vi "TempMeasOneSetZ.vi"(0 "meas_setting":T1 {"zStartDistCm" format="%.2f"; "numTxCycles" format="%.1f"; "profTxVoltageVolt" format="%#_1g"; "ceilTxVoltageVolt" format="%.2f"; "maxTxVoltageVolt" format="%.2f"; "focusRangeCm" format="%.1f"; "txFrequencyHz" format="%.2f"}, 1 "Comment(SN)":string, 2 "CW":bool, 5 "initial \ncommand":bool=TRUE, 7 "Database":T2, 9 "Z Address":T3, 11 "error in (no error)":errorcluster, 12 "Log file":path=path "nologfile") -> (15 "error out":errorcluster)   [LabVIEW 2016]
doc: "This program sets up runs one complete intensity measurement and voltage-dependent measurements. It calls subroutines to get hydrophone sensitivity, set Z system transmit parameters via Telnet, run the intensity measurement, and check the data. Next, the voltage-dependent measurement is made and checked. The data is saved to the database (or to a local file if errors have been found) and the results are printed. The program returns the result ID from the database, and any warnings or errors found."
uses:
  type def/ZAddress.ctl
  type def/Database.ctl
  type def/measSetting.ctl
  user/GrobaLimitVoltage.vi
  TemperatureMeasure/Thermal_type.vi
panel:
  in  "ScanRange coeff for PRF":dbl[][](array[numeric])=[[2.5, 1.6, 1.2, 1.0, 0.8], [2.3, 1.6, 1.2, 1.0, 0.8], [1.9, 1.6, 1.2, 1.0, 0.8], [1.7, 1.5, 1.2, 1.0, 0.8], [1.6, 1.4, 1.2, 1.0, 0.8]]
  out "Receive array":string[](array[string])=["\r\n220 OK\r\nContainers within Hardware Control Layer\r\n\tHardwareModel\r\n\tHardwareControl\r\n\tHardwareAlgorithm\r\n\tSeq\r\n\tBeamforming\r\n\tDigitalReceiver\r\n\tEchoProcessor\r\n\tFlowProcessor\r\n\tHardwareScanConverter\r\n\tSip\r\n\tVideoInterface\r\n\tRtc\r\n\tCine\r\nScalar Parameters of Hardware Control Layer\r\nArray Parameters of Hardware Control Layer\r\ndebug\tDebug Functions\r\nquit\tExit DIOS\r\nback\tPrevious menu\r\nmain\tTop menu\r\nhelp\tAvailable commands\r\n\r\n", "\r\n220 OK\r\nContainers within Beamforming\r\n\tCommon\r\n\tBImage\r\n\tCbImage\r\n\tDImage\r\nScalar Parameters of Beamforming\r\nArray Parameters of Beamforming\r\ndebug\tDebug Functions\r\nquit\tExit DIOS\r\nback\tPrevious menu\r\nmain\tTop menu\r\nhelp\tAvailable commands\r\n\r\n", "\r\n220 OK\r\nContainers within Common\r\nScalar Parameters of Common\r\n\tBfPropagationVelCmPerSec\t154000\r\n\tDisUnit\t0.00385\r\n\tHwRcInterruptMask\t63\r\n\tHwRcTVP\t3\r\n\tHwRxAac0\t175\r\n\tHwRxAac1\t0\r\n\tHwRxbfBlankingWord\t0\r\n\tHwRxbfCmd1Word\t4232\r\n\tHwRxbfCmd2Word\t2\r\n\tHwRxbf0Cmd2Word\t3\r\n\tHwRxbfStartDelayWord\t10\r\n\tHwTiAttenuatorSelect\t0\r\n\tHwTiBitEn\t25088\r\n\tHwTiDacCtrl0\t255\r\n\tHwTiDacCtrl1\t2303\r\n\tHwTiDacCtrl2\t3327\r\n\tHwTiDacCtrl3\t511\r\n\tHwTiDacCtrl4\t2559\r\n\tHwTiDacCtrl5\t3583\r\n\tHwTiDacCtrl6\t767\r\n\tHwTiDacCtrl7\t2815\r\n\tHwTiDacCtrl8\t3839\r\n\tHwTiDacCtrl9\t2047\r\n\tHwTiDacCtrl10\t4095\r\n\tHwTiDigitalDriveCtrl\t0\r\n\tHwTiDigitalInterruptPolarity\t0\r\n\tHwTiDigitalReadCtrl\t0\r\n\tHwTiEchoBoosterCtrl\t0\r\n\tHwTiGlobalCtrl\t1\r\n\tHwTiHighVoltEn\t0\r\n\tHwTiInterruptClear\t65535\r\n\tHwTiInterruptMask\t32767\r\n\tHwTiMiscBitCtrl\t12\r\n\tHwTiProbeSelect\t2\r\n\tHwTiTXCLTransfer\t0\r\n\tHwTiVoltMultiplexer\t0\r\n\tHwTrGlobalCtrlAll\t1\r\n\tHwTrGlobalCtrl0All\t0\r\n\tHwTrDiagnosticCtrlAll\t0\r\n\tHwTrInterruptMaskAll\t1\r\n\tHwTrInterruptClearAll\t1\r\n\tHwTrRealTimeCtrlAll\t40\r\n\tHwTrTgcAacSignalCtrlAll\t0\r\n\tRxDelayRefx\t1\r\n\tRxDelayRefy\t-1\r\n\tTrPartNumber\t5928150\r\n\tBfPropagationVelFactor\t1\r\n\tDigitizingRateHz\t4e+007\r\n\tHwRxBfVectorLengthWord\t0\r\n\tIsRxVectorLengthEn\t1\r\n\tNumChannels\t192\r\n\tProbeBandwidthHz\t3.6e+006\r\n\tProbeId\t171\r\n\tProbeNumElem\t192\r\n\tProbeNumRows\t1\r\n\tProbePitchCm\t0.02\r\n\tProbeRadiusElectricalCm\t0\r\n\tProbeType\t0\r\n\tPropagationVelCmPerSec\t154000\r\n\tRxApod2dEn\t0\r\n\tRxbfAdcDelayClocks\t10\r\n\tRxbfGainShift\t0\r\n\tRxDelayYOffsetSysClk4\t0\r\n\tTxPulserMaxVolt\t50\r\nArray Parameters of Common\r\n\tHwRxbf0AdGainA\tsize=64\r\n\tHwRxbf1AdGainA\tsize=64\r\n\tHwRxbf2AdGainA\tsize=64\r\n\tHwRxbf3AdGainA\tsize=64\r\n\tHwRxbf4AdGainA\tsize=64\r\n\tHwRxbf5AdGainA\tsize=64\r\n\tHwRxbf6AdGainA\tsize=64\r\n\tHwRxbf7AdGainA\tsize=64\r\n\tHwRxbf8AdGainA\tsize=64\r\n\tHwRxbf9AdGainA\tsize=64\r\n\tHwRxbf10AdGainA\tsize=64\r\n\tHwRxbf11AdGainA\tsize=64\r\n\tHwRxAdOffsetCalA\tsize=192\r\n\tHwRxApodFilterRamA\tsize=512\r\n\tHwRxbf0DelayCalA\tsize=64\r\n\tHwRxbf1DelayCalA\tsize=64\r\n\tHwRxbf2DelayCalA\tsize=64\r\n\tHwRxbf3DelayCalA\tsize=64\r\n\tHwRxbf4DelayCalA\tsize=64\r\n\tHwRxbf5DelayCalA\tsize=64\r\n\tHwRxbf6DelayCalA\tsize=64\r\n\tHwRxbf7DelayCalA\tsize=64\r\n\tHwRxbf8DelayCalA\tsize=64\r\n\tHwRxbf9DelayCalA\tsize=64\r\n\tHwRxbf10DelayCalA\tsize=64\r\n\tHwRxbf11DelayCalA\tsize=64\r\n\tHwRxbf0DxA\tsize=64\r\n\tHwRxbf1DxA\tsize=64\r\n\tHwRxbf2DxA\tsize=64\r\n\tHwRxbf3DxA\tsize=64\r\n\tHwRxbf4DxA\tsize=64\r\n\tHwRxbf5DxA\tsize=64\r\n\tHwRxbf6DxA\tsize=64\r\n\tHwRxbf7DxA\tsize=64\r\n\tHwRxbf8DxA\tsize=64\r\n\tHwRxbf9DxA\tsize=64\r\n\tHwRxbf10DxA\tsize=64\r\n\tHwRxbf11DxA\tsize=64\r\n\tHwRxbf0DyA\tsize=64\r\n\tHwRxbf1DyA\tsize=64\r\n\tHwRxbf2DyA\tsize=64\r\n\tHwRxbf3DyA\tsize=64\r\n\tHwRxbf4DyA\tsize=64\r\n\tHwRxbf5DyA\tsize=64\r\n\tHwRxbf6DyA\tsize=64\r\n\tHwRxbf7DyA\tsize=64\r\n\tHwRxbf8DyA\tsize=64\r\n\tHwRxbf9DyA\tsize=64\r\n\tHwRxbf10DyA\tsize=64\r\n\tHwRxbf11DyA\tsize=64\r\n\tHwRxbf0DzA\tsize=128\r\n\tHwRxbf1DzA\tsize=128\r\n\tHwRxbf2DzA\tsize=128\r\n\tHwRxbf3DzA\tsize=128\r\n\tHwRxbf4DzA\tsize=128\r\n\tHwRxbf5DzA\tsize=128\r\n\tHwRxbf6DzA\tsize=128\r\n\tHwRxbf7DzA\tsize=128\r\n\tHwRxbf8DzA\tsize=128\r\n\tHwRxbf9DzA\tsize=128\r\n\tHwRxbf10DzA\tsize=128\r\n\tHwRxbf11DzA\tsize=128\r\n\tHwRxbf0PosInApodWinA\tsize=64\r\n\tHwRxbf1PosInApodWinA\tsize=64\r\n\tHwRxbf2PosInApodWinA\tsize=64\r\n\tHwRxbf3PosInApodWinA\tsize=64\r\n\tHwRxbf4PosInApodWinA\tsize=64\r\n\tHwRxbf5PosInApodWinA\tsize=64\r\n\tHwRxbf6PosInApodWinA\tsize=64\r\n\tHwRxbf7PosInApodWinA\tsize=64\r\n\tHwRxbf8PosInApodWinA\tsize=64\r\n\tHwRxbf9PosInApodWinA\tsize=64\r\n\tHwRxbf10PosInApodWinA\tsize=64\r\n\tHwRxbf11PosInApodWinA\tsize=64\r\n\tHwRxMuxSelectLutA\tsize=512\r\n\tHwRxRamOffsetA\tsize=12\r\n\tHwTxDacA\tsize=2\r\n\tHwTxpgDelayAperA\tsize=393216\r\n\tNumBitsPerCycleA\tsize=49\r\n\tNumCyclesPerPassA\tsize=49\r\n\tNumWordsPerPassA\tsize=49\r\n\tRxAdGainA\tsize=256\r\n\tRxDelayCalA\tsize=768\r\n\tRxDxA\tsize=256\r\n\tRxDyA\tsize=256\r\n\tRxDzA\tsize=256\r\n\tRxMuxSelectLutPtrA\tsize=512\r\n\tRxPosInApodWinA\tsize=768\r\n\tTxDelayCalA\tsize=192\r\n\tTxpgWaveformHoutA\tsize=15680\r\n\tTxpgWaveformLoutA\tsize=15680\r\n\tYIndexTableA\tsize=256\r\n\tZIndexTableA\tsize=256\r\n\tInsertedProbeIdA\tsize=6\r\n\tPulseVoltageA\tsize=2\r\n\tRxApodFactorA\tsize=4\r\n\tRxApodSelA\tsize=4\r\n\tSysTxFreqHzA\tsize=49\r\ndebug\tDebug Functions\r\nquit\tExit DIOS\r\nback\tPrevious menu\r\nmain\tTop menu\r\nhelp\tAvailable commands\r\n\r\n", "220 OK\r\n", "250 20\r\n"]
  out "ProbeType":i8
  out "PID PRF":dbl format="%#.2f"
  out "error out 2":errorcluster caption="error out"
  out "size(s)":i32
  out "min Array":dbl[](array[numeric]) format="%.2f"
  out "Span Array":dbl[](array[numeric]) format="%.2f"
  out "TxElement array":i32[](array[numeric])
  out "Large RoiMin":dbl
  out "Large RoiSpan":dbl
  out "Small TxElement":i32
  in  "connection ID":refnum<k5>
  in  "tcp timeout (sec)":sgl=40.0 format="%.2f"
  in  "z tolCm":sgl=0.005 format="%.3f"
  # "Program constants"
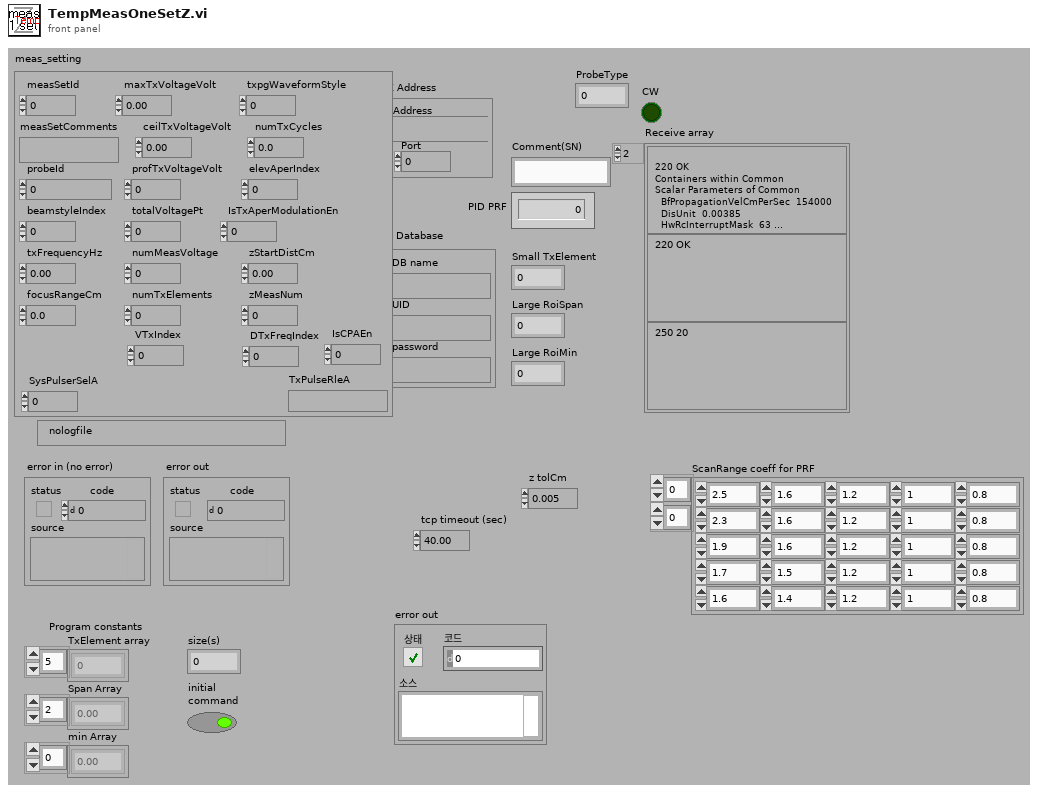
[diagram p1: front panel]
types:
  T1 = typedef "measSetting.ctl" = cluster{"measSetId":i32, "measSetComments":string, "probeId":sgl, "beamstyleIndex":i16, "txFrequencyHz":sgl, "focusRangeCm":sgl, "maxTxVoltageVolt":sgl, "ceilTxVoltageVolt":sgl, "profTxVoltageVolt":dbl, "totalVoltagePt":i8, "numMeasVoltage":i8, "numTxElements":i16, "txpgWaveformStyle":i8, "numTxCycles":sgl, "elevAperIndex":i8, "zStartDistCm":sgl, "zMeasNum":i8, "IsTxAperModulationEn":i8, "DTxFreqIndex":i16, "VTxIndex":i8, "IsCPAEn":i16, "SysPulserSelA":i16, "TxPulseRleA":string}
  T2 = typedef "Database.ctl" = cluster{"DB name":string, "UID":string, "password":string}
  T3 = typedef "ZAddress.ctl" = cluster{"Address":string, "Port":u16}
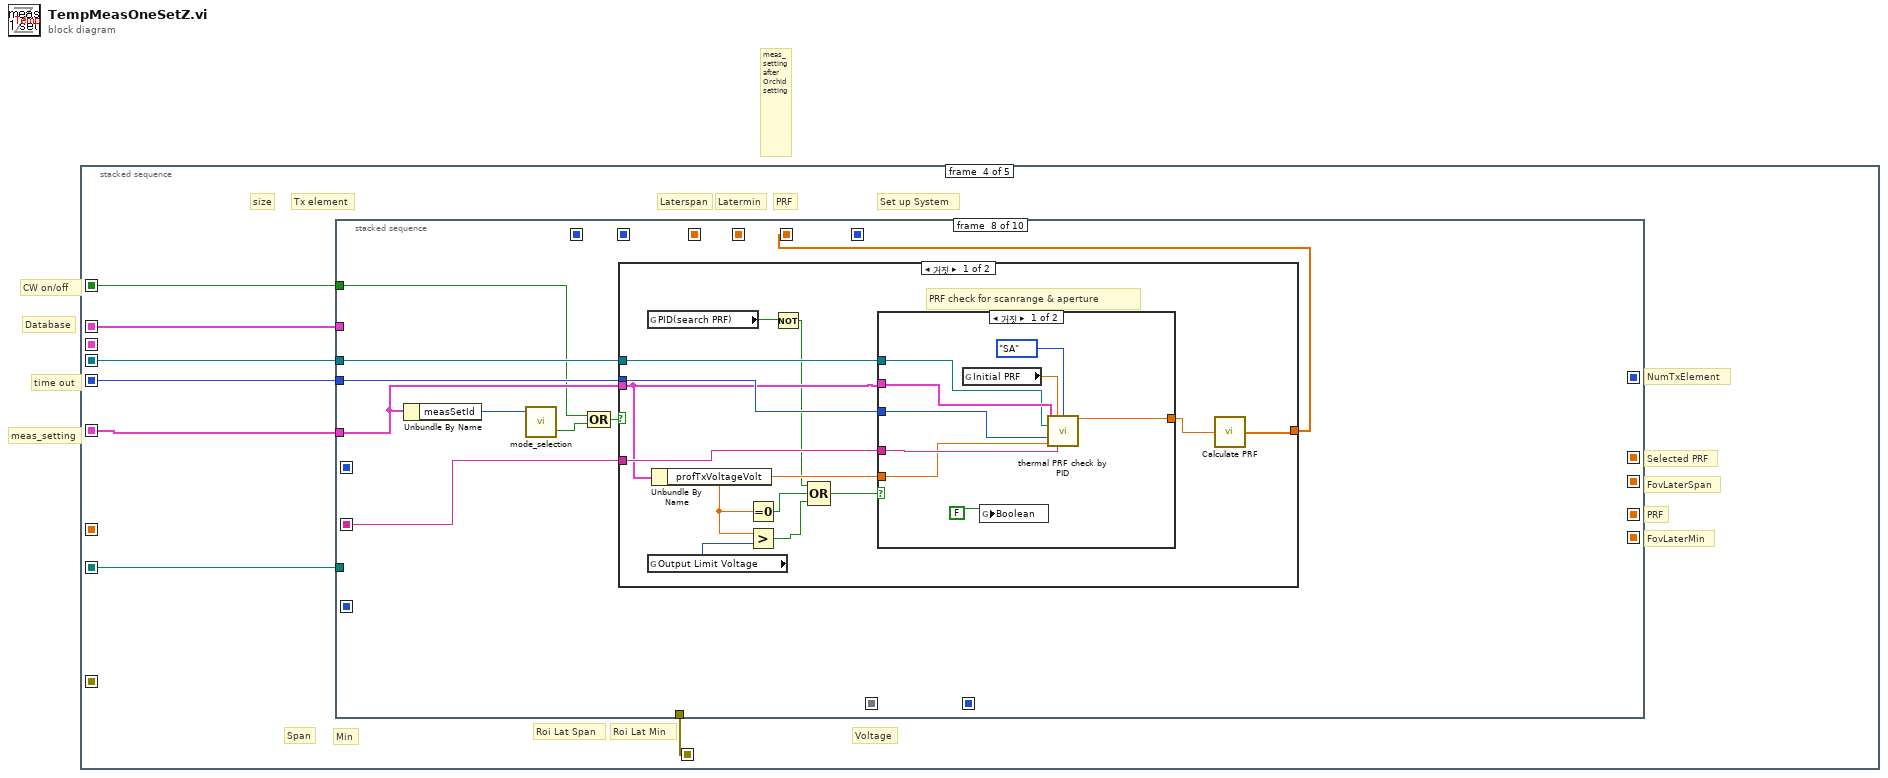
[diagram p0: block diagram]
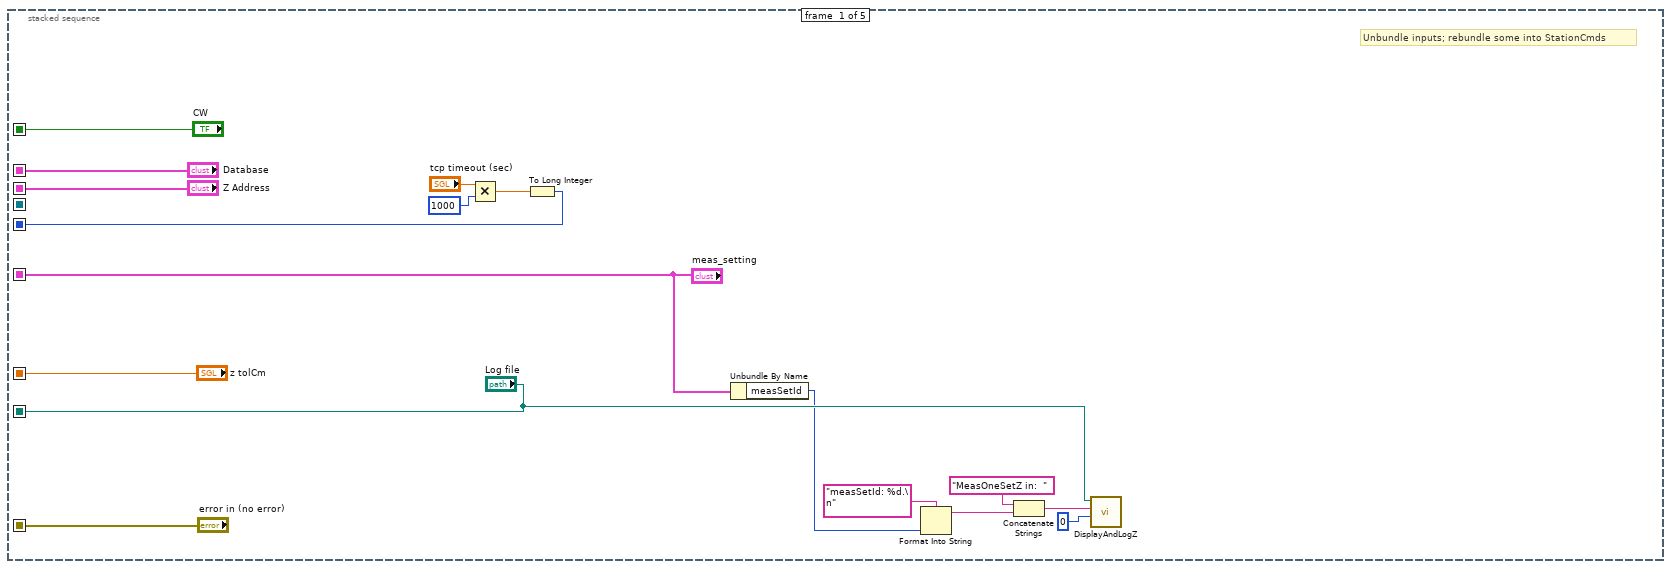
[diagram p2: hidden frame]
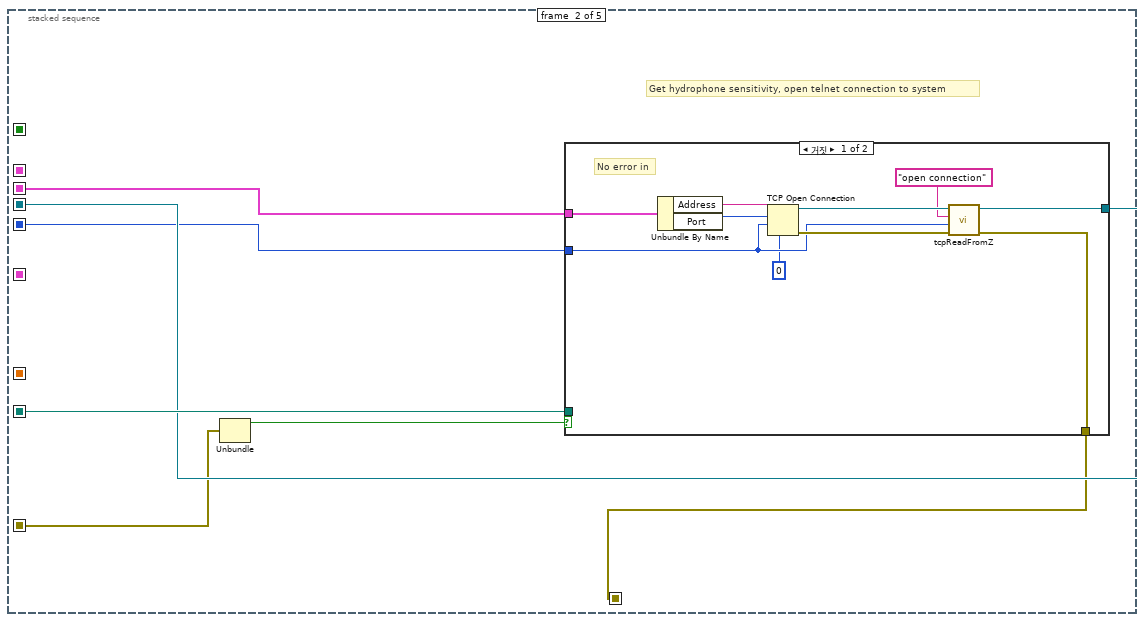
[diagram p3: hidden frame]
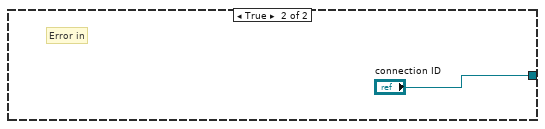
[diagram p4: hidden frame]
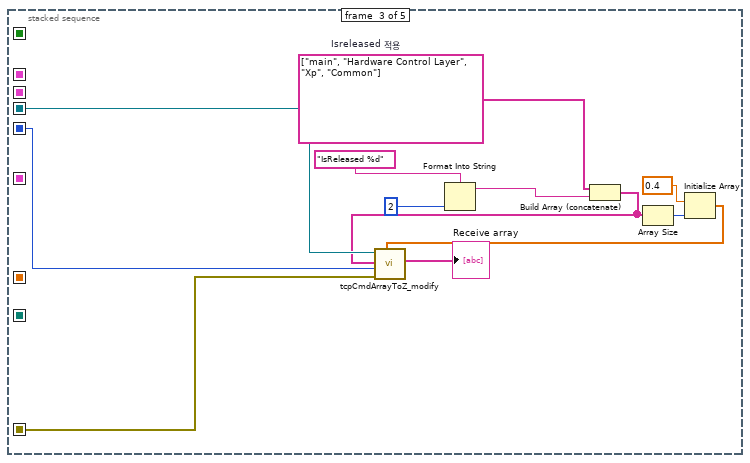
[diagram p5: hidden frame]
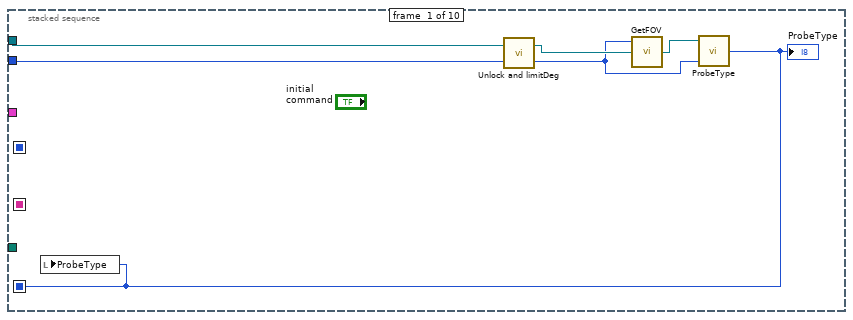
[diagram p6: hidden frame]
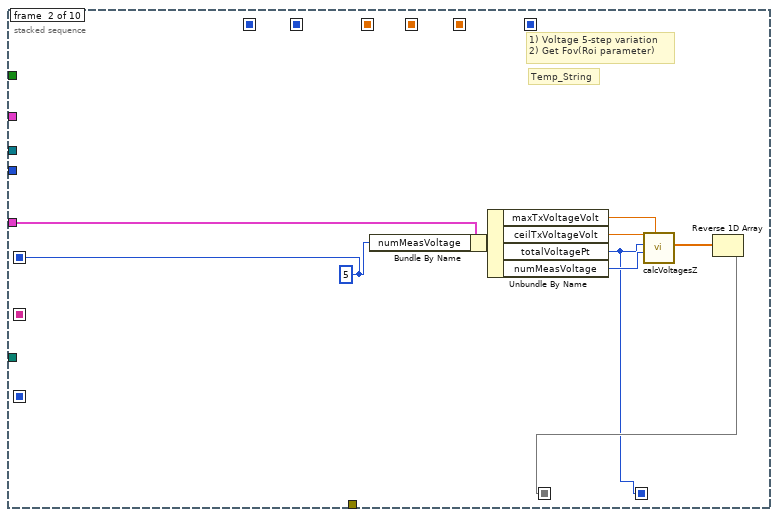
[diagram p7: hidden frame]
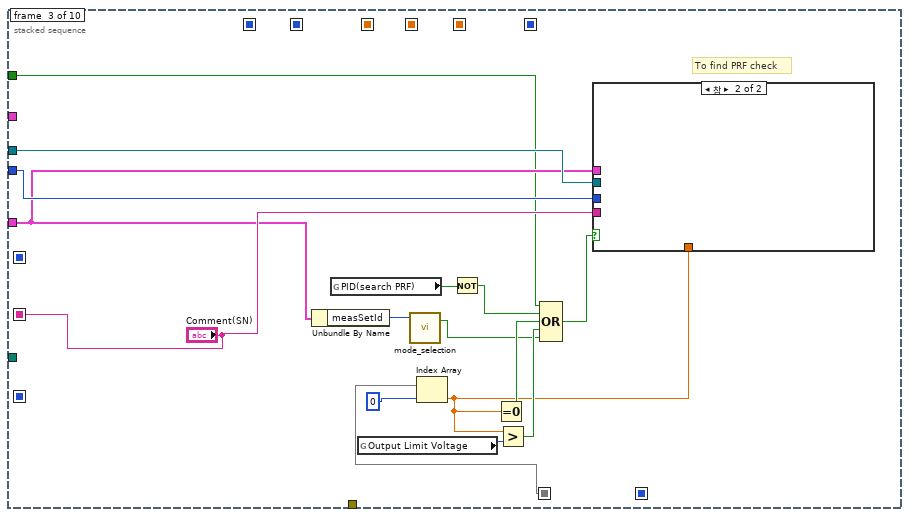
[diagram p8: hidden frame]
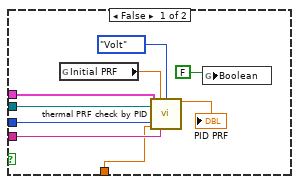
[diagram p9: hidden frame]
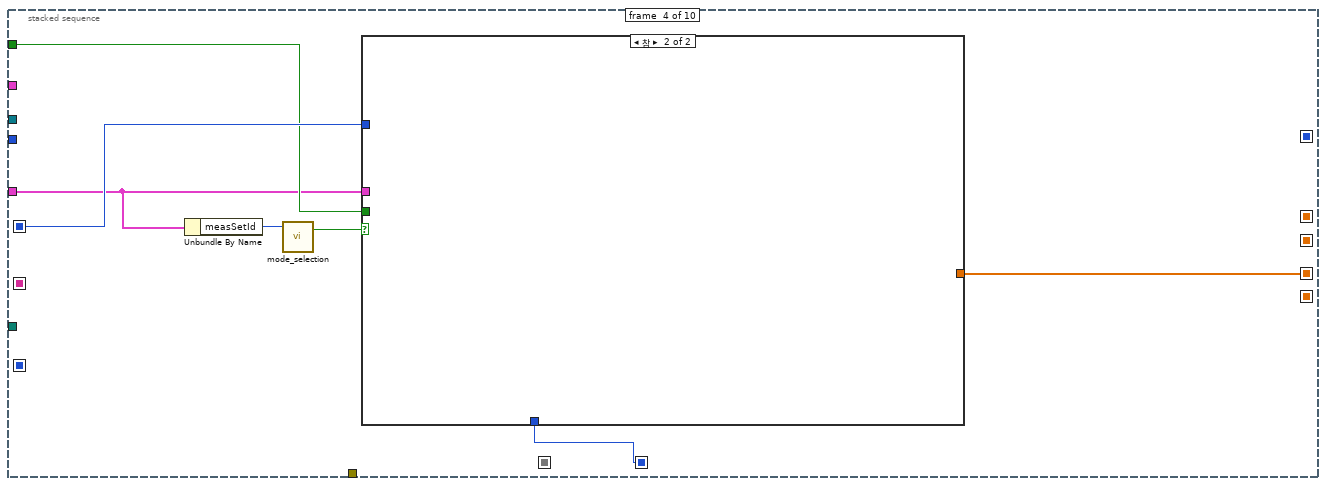
[diagram p10: hidden frame]
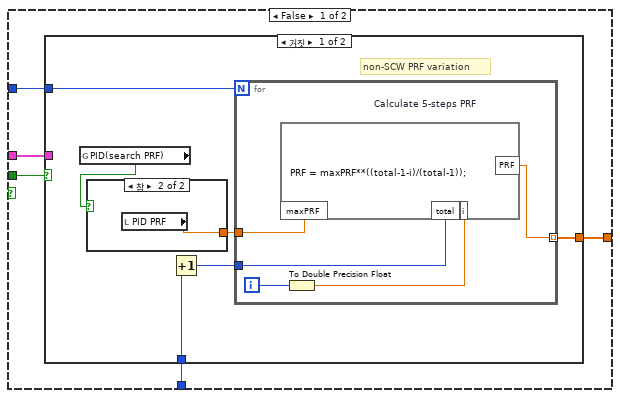
[diagram p11: hidden frame]
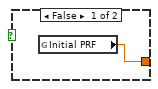
[diagram p12: hidden frame]
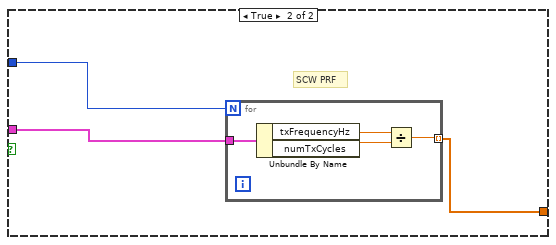
[diagram p13: hidden frame]
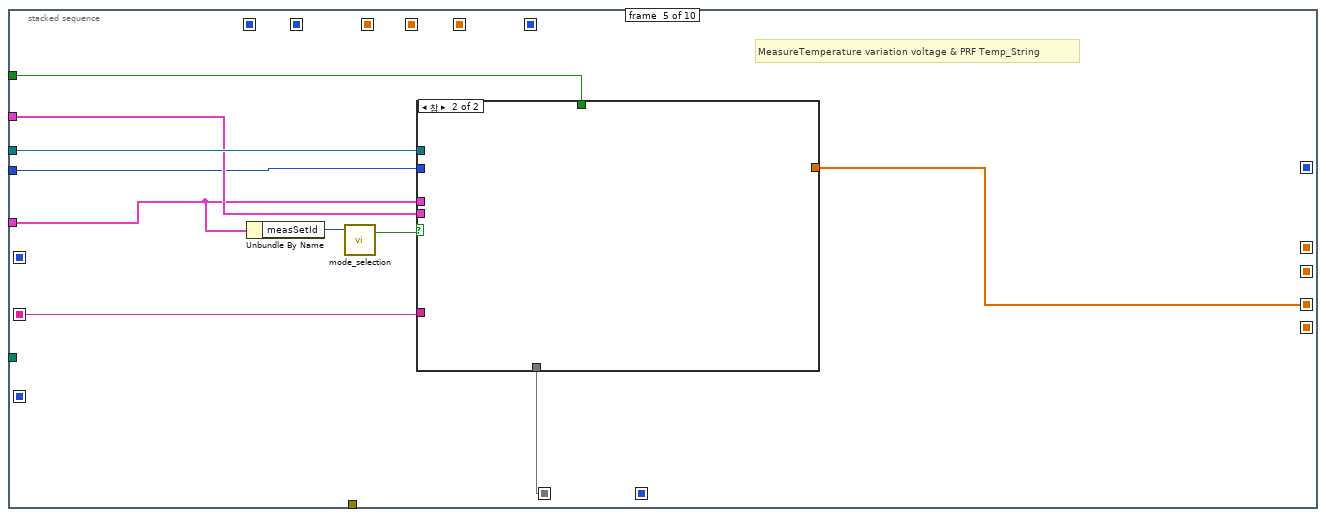
[diagram p14: hidden frame]
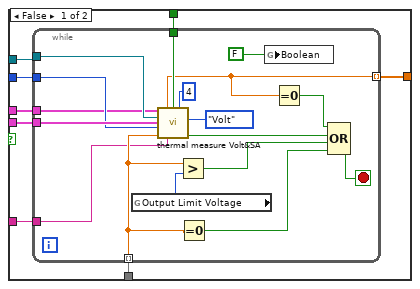
[diagram p15: hidden frame]
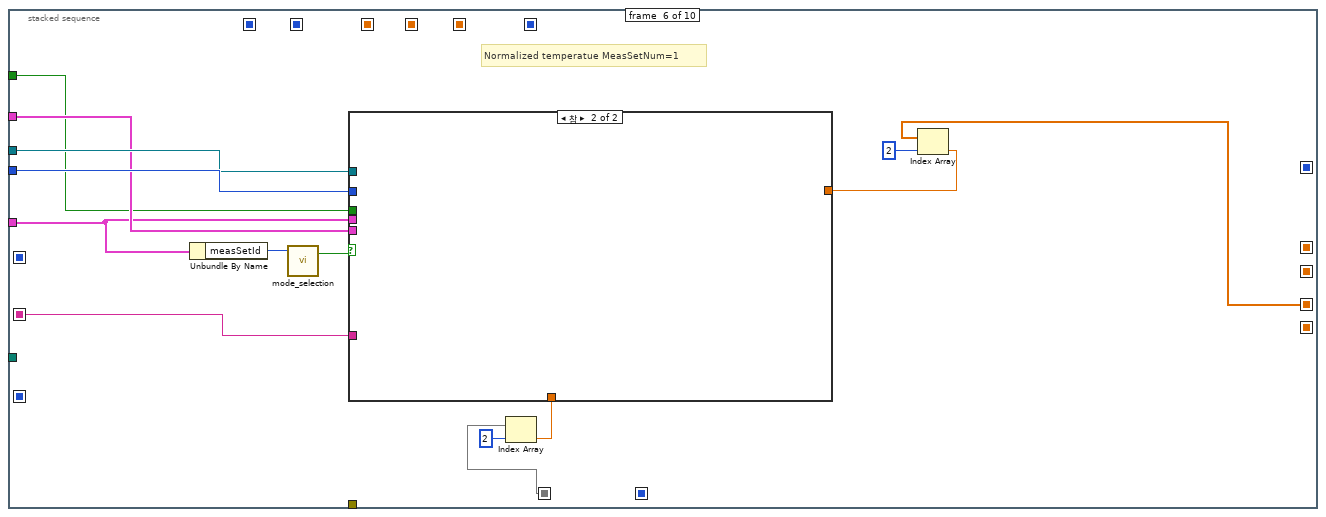
[diagram p16: hidden frame]
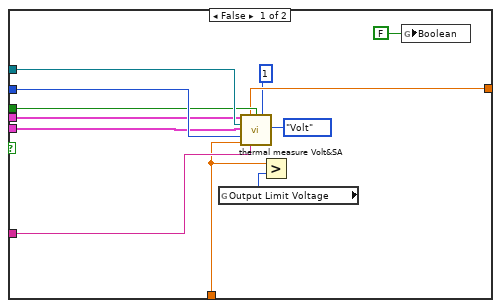
[diagram p17: hidden frame]
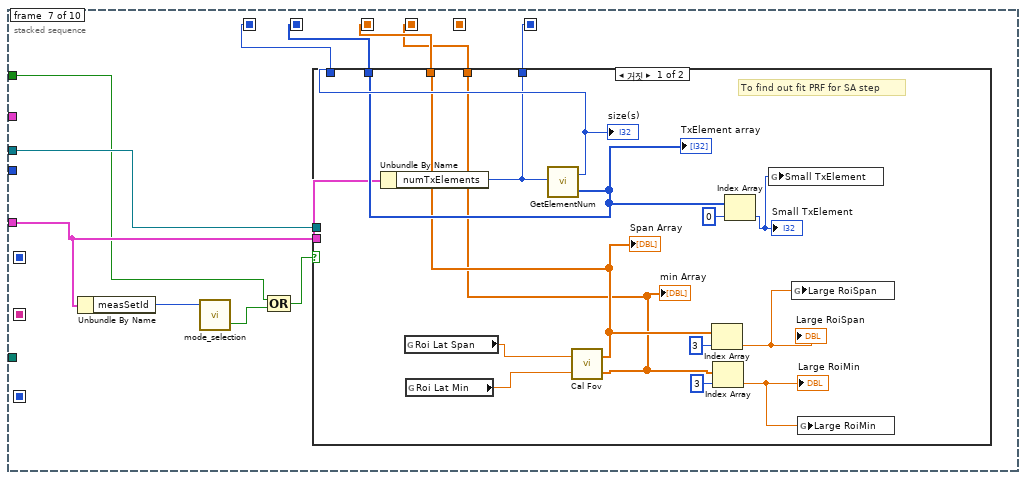
[diagram p18: hidden frame]
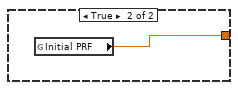
[diagram p20: hidden frame]
diagram:
  # "CW on/off"
  # "time out"
  # "Database"
  # "meas_setting"
  # "meas_setting\nafter Orchid setting"
  n1 = stacked-sequence {
    seq-local: ["Database" _ _ _ _] -> [_ _ _ w53 _]
    seq-local: ["Z Address" _ _ _ _] -> [_ w23 _ _ _]
    seq-local: ["Log file" _ _ _ _] -> [_ w24 _ w54 w372]
    seq-local: ["meas_setting" _ _ _ _] -> [_ _ _ w52 _]
    seq-local: ["z tolCm" _ _ _ _] -> [_ _ _ _ _]
    seq-local: [_ w21 _ _ _] -> [_ _ _ w48 w362]
    seq-local: [w5 _ _ _ _] -> [_ w20 w45 w50 w363]
    seq-local: [_ w22 _ _ _] -> [_ _ w47 w51 w364]
    seq-local: ["error in (no error)" _ _ _ _] -> [_ w19 w46 _ _]
    seq-local: ["CW" _ _ _ _] -> [_ _ _ w49 _]
    frame #0 {
      # "Unbundle inputs; rebundle some into StationCmds"
      n2 = Multiply(x="tcp timeout (sec)", y=i16 1000) -> (x*y=w6:sgl)
      n3 = To Long Integer(number=w6) -> (32bit integer=w5:i32)
      n4 = Unbundle By Name("meas_setting") -> ("measSetId"=w3:i32)
      n5 = Format Into String(format string="measSetId: %d.\n" ("Substring"), w3) -> (resulting string=w12:string)  [unwired: 2 in, 1 out]
      n6 = Concatenate Strings("MeasOneSetZ in:  " ("Substring"), w12) -> (w13:string)
      n7 = call "DisplayAndLogZ.vi"("Log file"="Log file", "message"=w13, "action (0: log+display)"=u16 0) -> ()  [unwired: 5 in, 1 out]
    }
    frame #1 {
      # "Get hydrophone sensitivity, open telnet connection to system"
      n8 = Unbundle(w19) -> ("status"=w18:bool)  [unwired: 2 out]
      n9 = case shown="거짓" w18 {
        tunnel: w24 -> [_ _]
        tunnel: w23 -> [w29 _]
        tunnel: [w28 "connection ID"] -> w22
        tunnel: [w26 _] -> w21
        tunnel: w20 -> [w27 _]
        frame False {
          # "No error in"
          n10 = Unbundle By Name(w29) -> ("Address"=w33:string, "Port"=w32:u16)
          n11 = TCP Open Connection(address=w33, remote port or service name=w32, timeout ms (60000)=w27, local port=u16 0) -> (connection ID=w31:refnum<k5>, error out=w34:errorcluster)  [unwired: 1 in]
          n12 = call "tcpReadFromZ.vi"("error in (no error)"=w34, "Timeout (40000 ms)"=w27, "Command sent"="open connection", "connection ID in"=w31) -> ("error out"=w26:errorcluster, "connection ID out"=w28:refnum<k5>)  [unwired: 3 in, 3 out]
        }
        frame True {
          # "Error in"
        }
      }
    }
    frame #2 {
      w38 = string[] ["main", "Hardware Control Layer", "Xp", "Common"]  # Isreleased 적용
      n13 = Format Into String(format string="IsReleased %d" ("Format String"), i16 2 ("입력 1")) -> (resulting string=w43:string)  [unwired: 2 in, 1 out]
      n14 = Build Array (concatenate)(w38, w43) -> (w40:string[])
      n15 = Array Size(array=w40) -> (size(s)=w42:i32)
      n16 = Initialize Array(0.4 ("element"), w42) -> (w39:dbl[])
      n17 = call "tcpCmdArrayToZ_modify.vi"("Delay (sec)"=w39, "error in (no error)"=w46, "Timeout (ms)"=w45, "Command array"=w40, "connection ID in"=w47) -> ("Receive array"=→"Receive array":string[])  [unwired: 2 in, 4 out]
    }
    frame #3 {
      # "Roi Lat Min"
      # "Roi Lat Span"
      # "Set up System"
      # "PRF"
      # "Latermin"
      # "Laterspan"
      # "Tx element"
      # "size"
      # "Selected PRF"
      # "Voltage"
      # "Span"
      # "Min"
      # "PRF"
      # "NumTxElement"
      # "FovLaterMin"
      # "FovLaterSpan"
      n18 = stacked-sequence {
        seq-local: [_ w62 _ _ _ _ _ _ _ _] -> [_ _ w84 _ w134 w175 _ _ _ _]
        seq-local: [_ _ _ w100 _ _ _ _ _ _] -> [_ _ _ _ w133 w174 _ _ _ w306]
        seq-local: [_ w64 _ _ _ _ _ _ _ _] -> [_ _ _ w101 _ _ _ _ _ _]
        seq-local: [_ _ _ _ _ _ _ _ w252 _] -> [_ _ _ _ _ _ _ _ _ w298]
        seq-local: [_ _ _ _ _ _ _ _ w259 _] -> [_ _ _ _ _ _ _ _ _ w305]
        seq-local: [_ _ _ _ _ _ _ _ w258 _] -> [_ _ _ _ _ _ _ _ _ w304]
        seq-local: [_ _ _ _ _ _ _ _ w251 _] -> [_ _ _ _ _ _ _ _ _ w303]
        seq-local: [_ _ "Comment(SN)" _ _ _ _ _ _ _] -> [_ _ _ _ w131 w170 _ w219 _ w307]
        seq-local: [_ _ _ _ _ _ w197 _ _ _] -> [_ _ _ _ _ _ _ _ w261 _]
        seq-local: [_ _ _ _ _ _ w196 _ _ _] -> [_ _ _ _ _ _ _ _ w260 _]
        seq-local: [_ _ _ _ _ _ w195 _ _ _] -> [_ _ _ _ _ _ _ _ w254 _]
        seq-local: [_ _ _ _ _ _ w194 _ _ _] -> [_ _ _ _ _ _ _ _ w253 _]
        seq-local: [_ _ _ _ _ _ _ w218 _ _] -> [_ _ _ _ _ _ _ _ w255 _]
        seq-local: [_ _ _ _ _ _ w191 _ _ _] -> [_ _ _ _ _ _ _ _ _ w301]
        seq-local: [_ w61 _ _ _ _ _ _ _ _] -> [_ _ _ w95 _ _ _ _ _ _]
        seq-local: [w58 _ _ _ _ _ _ _ _ _] -> [_ _ _ _ _ _ _ _ w245 w293]
        tunnel: w53 -> [_ _ _ _ w135 w171 _ _ _ w309]
        tunnel: w54 -> [_ _ _ _ _ _ _ _ _ _]
        tunnel: w52 -> [_ w67 w76 w97 w128 w163 w192 w216 w257 w302]
        tunnel: w51 -> [w60 _ w85 _ w136 w172 w198 w221 _ w308]
        tunnel: w50 -> [w59 _ w83 _ w132 w173 _ w220 _ w299]
        tunnel: w49 -> [_ _ w70 w99 w130 w169 w190 w214 w256 w300]
        tunnel: w48 -> [_ _ _ _ _ _ _ _ _ _]
        frame #0 {
          n19 = call "Unlock and limitDeg.vi"("Timeout (ms)"=w59, "connection ID in"=w60) -> ("Timeout (ms) 2"=w55:i32, "connection ID out"=w57:refnum<k5>)
          n20 = call "GetFOV.vi"("connection ID in"=w57, "Timeout (ms)"=w55) -> ("connection ID out"=w56:refnum<k5>)  [unwired: 1 in, 2 out]
          n21 = call "ProbeType.vi"("tcp timeout (ms)"=w55, "connection ID in"=w56) -> ("ProbeType"=w58:i8)  [unwired: 1 in]
          "ProbeType" <- w58
          n22 = local write "ProbeType"(w58) -> ()
        }
        frame #1 {
          w64 = i8 5 ("numMeasVoltage")
          # "Temp_String"
          # "1) Voltage 5-step variation\n2) Get Fov(Roi parameter)"
          n23 = Bundle By Name(cluster=w67, "numMeasVoltage"=w64) -> (w66:T1)
          n24 = Unbundle By Name(w66) -> ("maxTxVoltageVolt"=w65:sgl, "ceilTxVoltageVolt"=w69:sgl, "totalVoltagePt"=w61:i8, "numMeasVoltage"=w68:i8)
          n25 = call "calcVoltagesZ.vi"("maxTxVoltageVolt"=w65, "numMeasVoltage"=w68, "totalVoltagePt"=w61, "ceilTxVoltageVolt"=w69) -> ("Voltages"=w63:sgl[])  [unwired: 6 in]
          n26 = Reverse 1D Array(array=w63) -> (reversed array=w62:sgl[])
        }
        frame #2 {
          # "To find PRF check"
          n27 = Unbundle By Name(w76) -> ("measSetId"=w75:i32)
          n28 = global read "Thermal_type.vi" "PID(search PRF)"() -> (w73:bool)
          n29 = global read "GrobaLimitVoltage.vi" "Output Limit Voltage"() -> (w80:i16)
          n30 = call "mode_selection.vi"("MeasSetId"=w75) -> ("String_selection"=w74:bool)  [unwired: 3 in, 1 out]
          n31 = Index Array(array=w84, index=0) -> (element=w77:sgl)
          n32 = Not(x=w73) -> (.not. x?=w72:bool)
          n33 = Equal To 0?(x=w77) -> (x = 0?=w79:bool)
          n34 = Greater?(x=w77, y=w80) -> (0:w81:bool)
          n35 = Compound Arithmetic op=OR(w70, w72, w79, w81, w74) -> (w71:bool)
          n36 = case shown="참" w71 {
            tunnel: w85 -> [w94 _]
            tunnel: w83 -> [w93 _]
            tunnel: "Comment(SN)" -> [w92 _]
            tunnel: w76 -> [w91 _]
            tunnel: w77 -> [w90 _]
            frame False {
              n37 = global read "Thermal_type.vi" "Initial PRF"() -> (w89:dbl)
              n38 = call "thermal PRF check by PID.vi"("meas_setting"=w91, "PRF"=w89, "Measurement Type"=enum32{"Volt", "SA"}."Volt" ("PID Step"), "TCP from Orchid in"=w94, "tcp time out"=w93, "voltage"=w90, "Comment(SN)"=w92) -> ("PRF"=→"PID PRF":dbl)  [unwired: 6 in, 2 out]
              n39 = global write "GrobaLimitVoltage.vi" "Boolean"(FALSE) -> ()
            }
            frame True {
            }
          }
        }
        frame #3 {
          n40 = Unbundle By Name(w97) -> ("measSetId"=w98:i32)
          n41 = call "mode_selection.vi"("MeasSetId"=w98) -> ("String_selection"=w96:bool)  [unwired: 3 in, 1 out]
          n42 = case shown="참" w96 {
            tunnel: w101 -> [w106 _]
            tunnel: w97 -> [w105 _]
            tunnel: [w104 _] -> w100
            tunnel: w99 -> [w103 _]
            tunnel: w95 -> [w102 _]
            frame False {
              n43 = case shown="거짓" w103 {
                tunnel: w106 -> [w112 w121]
                tunnel: w105 -> [_ w122]
                tunnel: [w111 w120] -> w104
                tunnel: w102 -> [w107 _]
                frame False {
                  # "non-SCW PRF variation"
                  n44 = global read "Thermal_type.vi" "PID(search PRF)"() -> (w109:bool)
                  n45 = case shown="참" w109 {
                    tunnel: [w113 w114] -> w110
                    frame False {
                      n46 = global read "Thermal_type.vi" "Initial PRF"() -> (w113:dbl)
                    }
                    frame True {
                      n47 = local read "PID PRF"() -> (w114:dbl)
                    }
                  }
                  n48 = Increment(x=w107) -> (x+1=w108:i8)
                  n49 = for {
                    N: w112 -> [_]
                    tunnel: w110 -> [w119]
                    tunnel: w108 -> [w116]
                    tunnel: [w115] -> w111 mode=indexing
                    i -> [w117]
                    n50 = To Double Precision Float(number=w117) -> (double precision float=w118:dbl)
                    n51 = formula code="PRF = maxPRF**((total-1-i)/(total-1));" "Calculate 5-steps PRF"("total"=w116, "maxPRF"=w119, "i"=w118) -> ("PRF"=w115:dbl)
                  }
                }
                frame True {
                  # "SCW PRF"
                  n52 = for {
                    N: w121 -> [_]
                    tunnel: w122 -> [w126]
                    tunnel: [w123] -> w120 mode=indexing
                    n53 = Unbundle By Name(w126) -> ("txFrequencyHz"=w125:sgl, "numTxCycles"=w124:sgl)
                    n54 = Divide(x=w125, y=w124) -> (x/y=w123:sgl)
                  }
                }
              }
            }
            frame True {
            }
          }
        }
        frame #4 {
          # "MeasureTemperature variation voltage & PRF Temp_String"
          n55 = Unbundle By Name(w128) -> ("measSetId"=w129:i32)
          n56 = call "mode_selection.vi"("MeasSetId"=w129) -> ("String_selection"=w127:bool)  [unwired: 3 in, 1 out]
          n57 = case shown="참" w127 {
            tunnel: w136 -> [w144 _]
            tunnel: w135 -> [w143 _]
            tunnel: w134 -> [w142 _]
            tunnel: w133 -> [w141 _]
            tunnel: w132 -> [w140 _]
            tunnel: w131 -> [w139 _]
            tunnel: w128 -> [w138 _]
            tunnel: w130 -> [w137 _]
            frame False {
              n58 = while {
                tunnel: w142 -> [w152] mode=indexing
                tunnel: w144 -> [w161]
                tunnel: w143 -> [w160]
                tunnel: w141 -> [w148] mode=indexing
                tunnel: w140 -> [w154]
                tunnel: w139 -> [w151]
                tunnel: w138 -> [w150]
                tunnel: w137 -> [w149]
                stop <- w153 stop-if-true
                n59 = global read "GrobaLimitVoltage.vi" "Output Limit Voltage"() -> (w156:i16)
                n60 = call "thermal measure Volt&SA.vi"("meas_setting"=w150, "PRF"=w148, "CW"=w149, "measSetNum"=i16 4, "TCP from Orchid in"=w161, "Database"=w160, "Measurement Type"=enum32{"Volt", "SA"}."Volt", "tcp time out"=w154, "voltage"=w152, "Comment(SN)"=w151) -> ("Error(Volt & PRF)"=w158:bool)  [unwired: 4 in, 1 out]
                n61 = Greater?(x=w152, y=w156) -> (0:w159:bool)
                n62 = Equal To 0?(x=w152) -> (x = 0?=w155:bool)
                n63 = global write "GrobaLimitVoltage.vi" "Boolean"(FALSE) -> ()
                n64 = Equal To 0?(x=w148) -> (x = 0?=w147:bool)
                n65 = Compound Arithmetic op=OR(w147, w158, w159, w155) -> (w153:bool)
              }
            }
            frame True {
            }
          }
        }
        frame #5 {
          # "Normalized temperatue MeasSetNum=1"
          n66 = Unbundle By Name(w163) -> ("measSetId"=w164:i32)
          n67 = call "mode_selection.vi"("MeasSetId"=w164) -> ("String_selection"=w162:bool)  [unwired: 3 in, 1 out]
          n68 = Index Array(array=w175, index=2) -> (element=w167:sgl)
          n69 = Index Array(array=w174, index=2) -> (element=w166:dbl)
          n70 = case shown="참" w162 {
            tunnel: w173 -> [w187 _]
            tunnel: w172 -> [w186 _]
            tunnel: w171 -> [w185 _]
            tunnel: w170 -> [w184 _]
            tunnel: w163 -> [w183 _]
            tunnel: w169 -> [w182 _]
            tunnel: w167 -> [w181 _]
            tunnel: w166 -> [w180 _]
            frame False {
              n71 = global read "GrobaLimitVoltage.vi" "Output Limit Voltage"() -> (w178:i16)
              n72 = call "thermal measure Volt&SA.vi"("meas_setting"=w183, "PRF"=w180, "CW"=w182, "measSetNum"=i16 1, "TCP from Orchid in"=w186, "Database"=w185, "Measurement Type"=enum32{"Volt", "SA"}."Volt", "tcp time out"=w187, "voltage"=w181, "Comment(SN)"=w184) -> ()  [unwired: 4 in, 2 out]
              n73 = Greater?(x=w181, y=w178) -> ()  [unwired: 1 out]
              n74 = global write "GrobaLimitVoltage.vi" "Boolean"(FALSE) -> ()
            }
            frame True {
            }
          }
        }
        frame #6 {
          n75 = Unbundle By Name(w192) -> ("measSetId"=w193:i32)
          n76 = call "mode_selection.vi"("MeasSetId"=w193) -> ("Coeff_selection"=w189:bool)  [unwired: 3 in, 1 out]
          n77 = Compound Arithmetic op=OR(w190, w189) -> (w188:bool)
          n78 = case shown="거짓" w188 {
            tunnel: w198 -> [_ _]
            tunnel: [w212 _] -> w197
            tunnel: [w211 _] -> w196
            tunnel: [w210 _] -> w195
            tunnel: [w209 _] -> w194
            tunnel: w192 -> [w208 _]
            tunnel: [w207 _] -> w191
            frame False {
              # "To find out fit PRF for SA step"
              n79 = Unbundle By Name(w208) -> ("numTxElements"=w207:i16)
              n80 = global read "Thermal_type.vi" "Roi Lat Span"() -> (w200:dbl)
              n81 = global read "Thermal_type.vi" "Roi Lat Min"() -> (w199:dbl)
              n82 = call "GetElementNum.vi"("input variable"=w207) -> ("size(s)"=w212:i32, "appended array"=w211:i32[])
              "TxElement array" <- w211
              "size(s)" <- w212
              n83 = call "Cal Fov.vi"("min"=w199, "Span"=w200) -> ("min"=w209:dbl[], "Span"=w210:dbl[])
              "Span Array" <- w210
              "min Array" <- w209
              n84 = Index Array(array=w210, index=3) -> (element=w202:dbl)
              "Large RoiSpan" <- w202
              n85 = Index Array(array=w209, index=3) -> (element=w201:dbl)
              "Large RoiMin" <- w201
              n86 = Index Array(array=w211, index=0) -> (element=w206:i32)
              "Small TxElement" <- w206
              n87 = global write "Thermal_type.vi" "Small TxElement"(w206) -> ()
              n88 = global write "Thermal_type.vi" "Large RoiSpan"(w202) -> ()
              n89 = global write "Thermal_type.vi" "Large RoiMin"(w201) -> ()
            }
            frame True {
            }
          }
        }
        frame #7 {
          n90 = Unbundle By Name(w216) -> ("measSetId"=w217:i32)
          n91 = call "mode_selection.vi"("MeasSetId"=w217) -> ("Coeff_selection"=w215:bool)  [unwired: 3 in, 1 out]
          n92 = Compound Arithmetic op=OR(w214, w215) -> (w213:bool)
          n93 = case shown="거짓" w213 {
            tunnel: w221 -> [w234 _]
            tunnel: w220 -> [w233 _]
            tunnel: w219 -> [w232 _]
            tunnel: w216 -> [w227 _]
            tunnel: [w222 _] -> w218
            frame False {
              # "PRF check for scanrange & aperture"
              n94 = global read "Thermal_type.vi" "PID(search PRF)"() -> (w225:bool)
              n95 = global read "GrobaLimitVoltage.vi" "Output Limit Voltage"() -> (w230:i16)
              n96 = Unbundle By Name(w227) -> ("profTxVoltageVolt"=w226:dbl)
              n97 = Equal To 0?(x=w226) -> (x = 0?=w229:bool)
              n98 = Greater?(x=w226, y=w230) -> (0:w231:bool)
              n99 = Not(x=w225) -> (.not. x?=w224:bool)
              n100 = Compound Arithmetic op=OR(w224, w229, w231) -> (w228:bool)
              n101 = case shown="거짓" w228 {
                tunnel: w234 -> [w239 _]
                tunnel: w233 -> [w243 _]
                tunnel: w232 -> [w242 _]
                tunnel: w227 -> [w241 _]
                tunnel: w226 -> [w240 _]
                tunnel: [w235 w244] -> w223
                frame False {
                  n102 = global read "Thermal_type.vi" "Initial PRF"() -> (w237:dbl)
                  n103 = global write "GrobaLimitVoltage.vi" "Boolean"(FALSE) -> ()
                  n104 = call "thermal PRF check by PID.vi"("meas_setting"=w241, "PRF"=w237, "Measurement Type"=enum32{"Volt", "SA"}."SA" ("PID Step"), "TCP from Orchid in"=w239, "tcp time out"=w243, "voltage"=w240, "Comment(SN)"=w242) -> ("PRF"=w235:dbl)  [unwired: 6 in, 2 out]
                }
                frame True {
                  n105 = global read "Thermal_type.vi" "Initial PRF"() -> (w244:dbl)
                }
              }
              n106 = call "Calculate PRF.vi"("PRF"=w223) -> ("PRF Array"=w222:dbl[])
            }
            frame True {
            }
          }
        }
        frame #8 {
          # "To create Tx element * scanrange(16ea) variation"
          n107 = Unbundle By Name(w257) -> ("measSetId"=w250:i32)
          n108 = call "mode_selection.vi"("MeasSetId"=w250) -> ("Coeff_selection"=w248:bool)  [unwired: 3 in, 1 out]
          n109 = Compound Arithmetic op=OR(w256, w248) -> (w249:bool)
          n110 = case shown="1" w245 {
            tunnel: w253 -> [w262 w265]
            tunnel: w254 -> [w263 w269]
            tunnel: [w263 w268] -> w247
            tunnel: [w262 w264] -> w246
            frame 0, Default {
            }
            frame 1 {
              n111 = Delete From Array(array=w269, length=3 ("인덱스"), index=1 ("길이")) -> (array with subset deleted=w268:dbl[])  [unwired: 1 out]
              n112 = Delete From Array(array=w265, length=3 ("인덱스"), index=1 ("길이")) -> (array with subset deleted=w264:dbl[])  [unwired: 1 out]
            }
          }
          n113 = case shown="거짓" w249 {
            tunnel: w261 -> [w280 _]
            tunnel: w260 -> [w279 _]
            tunnel: [w278 _] -> w259
            tunnel: w247 -> [w277 _]
            tunnel: w246 -> [w276 _]
            tunnel: [w275 _] -> w258
            tunnel: [w274 _] -> w251
            tunnel: w255 -> [w272 _]
            tunnel: [w273 _] -> w252
            frame False {
              n114 = for {
                N: w280 -> [_]
                tunnel: w279 -> [w288] mode=indexing
                tunnel: [w287] -> w278 mode=indexing
                tunnel: w277 -> [w286]
                tunnel: w276 -> [w285]
                tunnel: [w284] -> w275 mode=indexing
                tunnel: [w283] -> w274 mode=indexing
                tunnel: [w282] -> w273 mode=indexing
                tunnel: w272 -> [w281] mode=indexing
                n115 = for {
                  tunnel: w288 -> [w292]
                  tunnel: [w292] -> w287 mode=indexing
                  tunnel: w286 -> [w291] mode=indexing
                  tunnel: w285 -> [w290] mode=indexing
                  tunnel: [w291] -> w284 mode=indexing
                  tunnel: [w290] -> w283 mode=indexing
                  tunnel: w281 -> [w289]
                  tunnel: [w289] -> w282 mode=indexing
                }
              }
            }
            frame True {
            }
          }
        }
        frame #9 {
          n116 = Unbundle By Name(w302) -> ("measSetId"=w297:i32)
          n117 = call "mode_selection.vi"("MeasSetId"=w297) -> ("Coeff_selection"=w296:bool)  [unwired: 3 in, 1 out]
          n118 = Compound Arithmetic op=OR(w300, w296) -> (w295:bool)
          n119 = case shown="0, 기본" w293 {
            tunnel: w298 -> [w360 w361]
            tunnel: [w359 w361] -> w294
            frame 0, Default {
              n120 = Divide(x=w360, y="ScanRange coeff for PRF") -> (x/y=w359:dbl[][])
            }
            frame 1 {
            }
          }
          n121 = case shown="거짓" w295 {
            tunnel: w309 -> [w319 _]
            tunnel: w302 -> [w318 _]
            tunnel: w308 -> [w317 _]
            tunnel: w307 -> [w316 _]
            tunnel: w306 -> [_ _]
            tunnel: w305 -> [w315 _]
            tunnel: w294 -> [w314 _]
            tunnel: w304 -> [w313 _]
            tunnel: w303 -> [w312 _]
            tunnel: w301 -> [w311 _]
            tunnel: w299 -> [w310 _]
            frame False {
              # "16ea Scanrange * Aperture"
              n122 = for {
                tunnel: w319 -> [w329]
                tunnel: w318 -> [w328]
                tunnel: w317 -> [w327]
                tunnel: w316 -> [w326]
                tunnel: w315 -> [w325] mode=indexing
                tunnel: w314 -> [w324] mode=indexing
                tunnel: w313 -> [w323] mode=indexing
                tunnel: w312 -> [w322] mode=indexing
                tunnel: w311 -> [w321]
                tunnel: w310 -> [w320]
                n123 = while {
                  tunnel: w329 -> [w343]
                  tunnel: w328 -> [w342]
                  tunnel: w327 -> [w341]
                  tunnel: w326 -> [w339]
                  tunnel: w325 -> [w338] mode=indexing
                  tunnel: w324 -> [w337] mode=indexing
                  tunnel: w323 -> [w335] mode=indexing
                  tunnel: w322 -> [w336] mode=indexing
                  tunnel: w321 -> [w334]
                  tunnel: w320 -> [w330]
                  stop <- w333 stop-if-true
                  n124 = Equal To 0?(x=w335) -> (x = 0?=w331:bool)
                  n125 = Equal To 0?(x=w338) -> (x = 0?=w332:bool)
                  n126 = Compound Arithmetic op=OR(w331, w332) -> (w333:bool)
                  n127 = Unbundle By Name(w342) -> ("profTxVoltageVolt"=w340:dbl)
                  n128 = case shown="참" w333 {
                    tunnel: w343 -> [w357 _]
                    tunnel: w342 -> [w356 _]
                    tunnel: w341 -> [w355 _]
                    tunnel: w340 -> [w354 _]
                    tunnel: w339 -> [w353 _]
                    tunnel: w338 -> [w352 _]
                    tunnel: w337 -> [w351 _]
                    tunnel: w336 -> [w350 _]
                    tunnel: w335 -> [w349 _]
                    tunnel: w334 -> [w348 _]
                    tunnel: w330 -> [w345 _]
                    frame False {
                      n129 = call "thermal measure Volt&SA.vi"("meas_setting"=w356, "PRF"=w351, "CW"=FALSE, "measSetNum"=i16 3, "RoiLaterMin"=w350, "TCP from Orchid in"=w355, "RoiLateralSpan"=w349, "Database"=w357, "Measurement Type"=enum32{"Volt", "SA"}."SA", "tcp time out"=w345, "voltage"=w354, "Comment(SN)"=w353, "Entire_element"=w348, "NumTxElement"=w352) -> ()  [unwired: 2 out]
                    }
                    frame True {
                    }
                  }
                }
              }
            }
            frame True {
            }
          }
        }
      }
    }
    frame #4 {
      n130 = stacked-sequence {
        tunnel: w364 -> [w375 w381]
        tunnel: w363 -> [w374 w380]
        frame #0 {
          n131 = case shown="거짓" FALSE {
            tunnel: w375 -> [_ w377]
            tunnel: w374 -> [_ w376]
            frame False {
            }
            frame True {
              w378 = string[] ["main", "debug", "Ic", "Ic Events", "Common Events", "FreezeEvent"]  # Tx voltage change
              w379 = sgl[] [0.0, 0.0, 0.0, 0.0, 0.0, 1.0]  # Delay (sec)
              n132 = call "tcpCmdArrayToZ_modify.vi"("Delay (sec)"=w379, "Timeout (ms)"=w376, "Command array"=w378, "connection ID in"=w377) -> ()  [unwired: 3 in, 5 out]
            }
          }
        }
        frame #1 {
          # "Close telnet connection, write log"
          # "write \"quit\" even\nif error exists"
          n133 = TCP Write(connection ID=w381, data in="quit\n", 9:w380) -> (connection ID out=w382:refnum<k5>, error out=w384:errorcluster)  [unwired: 1 in, 1 out]
          n134 = TCP Close Connection(connection ID=w382, error in (no error)=w384) -> (error out=→"error out":errorcluster)  [unwired: 1 in, 1 out]
        }
      }
      n135 = Get Date/Time String() -> (date string=w370:string, time string=w368:string)  [unwired: 3 in]
      n136 = Concatenate Strings("MeasOneSetZ out: " ("Substring"), w370, "  ", w368, "\n" ("Substring")) -> (w366:string)
      n137 = call "DisplayAndLogZ.vi"("Log file"=w372, "message"=w366, "action (0: log+display)"=u16 0) -> ()  [unwired: 5 in, 1 out]
      "error out 2" <- w362
    }
  }
